vi "Run_7_of_X_Tests.vi"() -> ()   [LabVIEW 2019]
uses:
  <vilib>/Rock Robotics/WPI/ThirdParty/JAS_Junk/TrajLib/Trajectory_Library.lvlib
panel:
  out "Diff Drive Pose Est 2":bool
  out "Coordinate System":bool
  out "String":string
  out "DC Motor Simulation":bool
  out "Debounce":bool
  out "All Tests Finished":bool
  out "Diff Drive Pose Est":bool
  # "FORMAL TRAJECTORY / CONTROL LIBRARY TEST PROCEDURE"
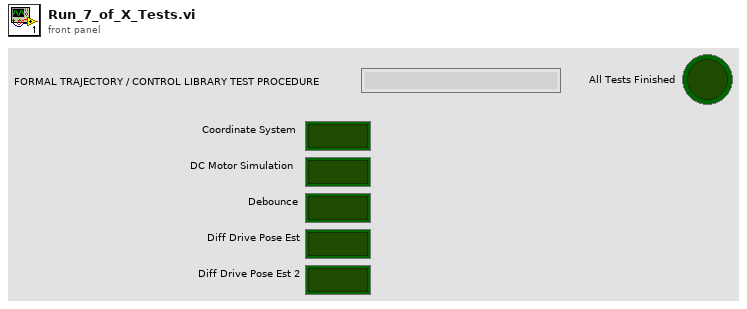
[diagram p1: front panel]
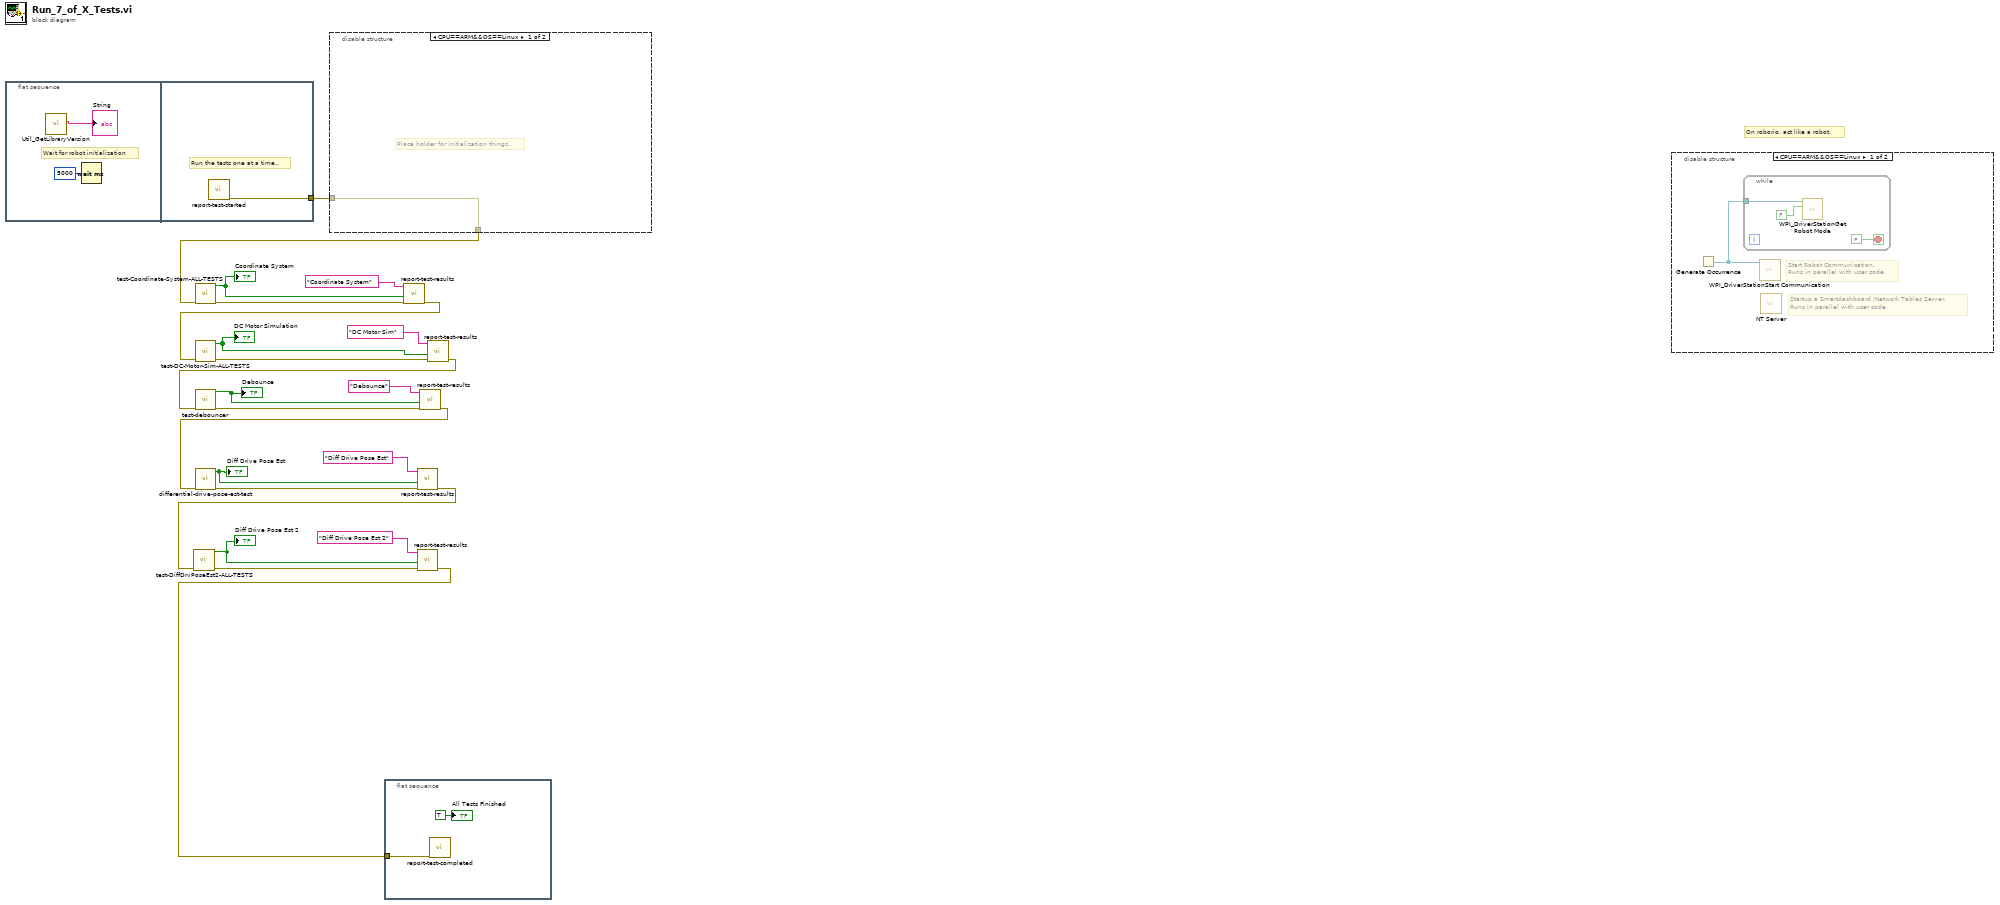
[diagram p0: block diagram]
diagram:
  # "On roborio, act like a robot."
  n1 = flat-sequence {
    tunnel: [w25] -> w16
    frame #0 {
      # "Wait for robot initialization"
      n2 = call <vilib>:"Util_GetLibraryVersion.vi"() -> ("TrajLibVersion"=→"String":string)  [unwired: 11 in]
      n3 = Wait (ms)(milliseconds to wait=u32 5000) -> ()  [unwired: 1 out]
    }
    frame #1 {
      # "Run the tests one at a time.."
      n4 = call "report-test-started.vi"() -> ("error out"=w25:errorcluster)  [unwired: 11 in]
    }
  }
  n5 = disable-structure shown="CPU==ARM&&OS==Linux" {
    disable-tunnel: w16 -> [w26 w27]
    disable-tunnel: [w26 w27] -> w7
    frame condition #0 {
      # "Place holder for initialization things."
    }
    frame condition #1 (active) {
    }
  }
  n6 = call "test-Coordinate-System-ALL-TESTS.vi"("error in (no error)"=w7) -> ("error out"=w9:errorcluster, "All Passed"=w8:bool)  [unwired: 9 in]
  "Coordinate System" <- w8
  n7 = flat-sequence {
    tunnel: w1 -> [w28]
    frame #0 {
      n8 = call "report-test-completed.vi"("error in (no error)"=w28) -> ()  [unwired: 10 in, 1 out]
      "All Tests Finished" <- TRUE ("All Tests Finished")
    }
  }
  n9 = call "report-test-results.vi"("error in (no error)"=w9, "TestPassed"=w8, "Test Name"="Coordinate System") -> ("error out"=w6:errorcluster)  [unwired: 8 in]
  n10 = call "test-DC-Motor-Sim-ALL-TESTS.vi"("error in (no error)"=w6) -> ("error out"=w14:errorcluster, "All Passed"=w13:bool)  [unwired: 9 in]
  "DC Motor Simulation" <- w13
  n11 = call "report-test-results.vi"("error in (no error)"=w14, "TestPassed"=w13, "Test Name"="DC Motor Sim") -> ("error out"=w12:errorcluster)  [unwired: 8 in]
  n12 = call "test-debouncer.vi"("error in (no error)"=w12) -> ("error out"=w18:errorcluster, "ALL TESTS PASSED"=w21:bool)  [unwired: 9 in]
  "Debounce" <- w21
  n13 = call "report-test-results.vi"("error in (no error)"=w18, "TestPassed"=w21, "Test Name"="Debounce") -> ("error out"=w11:errorcluster)  [unwired: 8 in]
  n14 = call "differential-drive-pose-est-test.vi"("error in (no error)"=w11) -> ("error out"=w17:errorcluster, "Test Passed"=w19:bool)  [unwired: 9 in]
  "Diff Drive Pose Est" <- w19
  n15 = call "report-test-results.vi"("error in (no error)"=w17, "TestPassed"=w19, "Test Name"="Diff Drive Pose Est") -> ("error out"=w4:errorcluster)  [unwired: 8 in]
  n16 = call "test-DiffDrvPoseEst2-ALL-TESTS.vi"("error in (no error)"=w4) -> ("error out"=w3:errorcluster, "All Passed"=w2:bool)  [unwired: 9 in]
  "Diff Drive Pose Est 2" <- w2
  n17 = call "report-test-results.vi"("error in (no error)"=w3, "TestPassed"=w2, "Test Name"="Diff Drive Pose Est 2") -> ("error out"=w1:errorcluster)  [unwired: 8 in]
  n18 = disable-structure shown="CPU==ARM&&OS==Linux" {
    frame condition #0 {
      # "Startup a Smartdashboard /Network Tables Server.\nRuns in parallel with user code."
      # "Start Robot Communication.\nRuns in parallel with user code."
      n19 = Generate Occurrence() -> (w30:refnum<k4>)
      n20 = while {
        tunnel: w30 -> [w33]
        stop <- FALSE stop-if-true
        n21 = call <vilib>:"WPI_DriverStationGet Robot Mode.vi"("Finish"=FALSE, "DS Occurrence"=w33) -> ()  [unwired: 10 out]
      }
      n22 = call <vilib>:"WPI_DriverStationStart Communication.vi"("occurrence"=w30) -> ()  [unwired: 2 in, 9 out]
      n23 = call <vilib>:"NT Server.vi"() -> ()  [unwired: 12 in]
    }
    frame condition #1 (active) {
    }
  }
